vi "Result.vi"(8 "error in (no error)":errorcluster, 10 "Result":T1={"Name"="", "Message"="", "Description"="", "Status"=enum."Passed", "Result Type"=enum."Case", "Execution Time"=0.0}, 11 "Test Result Tree V2 in":refnum<class "Test Result Tree V2.lvclass">) -> (0 "error out":errorcluster)   [LabVIEW 2020, in "Test Result Tree V2.lvclass"]
uses:
  Test Result Tree V2.lvclass
  C:/Git/astemes-lunit/source/Rewrite Project/Deprecated/Test Tree/Test Tree.lvclass
  Result/Result.ctl
  Result/Status.ctl
  Result/Type.ctl
  Test Tree/Test Tree.lvclass/Test Tree.ctl
  Utilities/Status to Glyph.vi
  Test Tree/Test Tree.lvclass
  Result/Result.lvlib
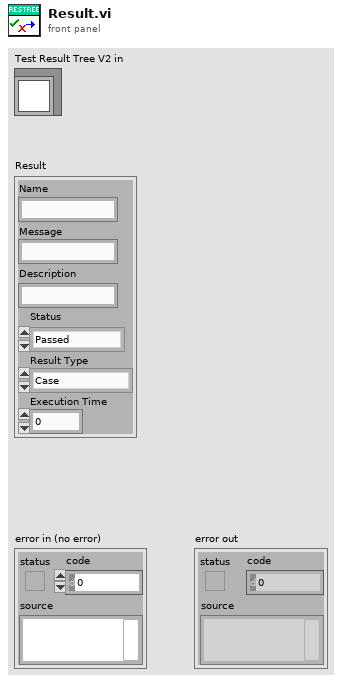
[diagram p1: front panel]
types:
  T1 = typedef "Result.lvlib/Result.ctl" = cluster{"Name":string, "Message":string, "Description":string, "Status":T2, "Result Type":T3, "Execution Time":dbl}
  T2 = typedef "Result.lvlib/Status.ctl" = enum16{"", "Passed", "Failed", "Error", "Skipped", "Setup Error", "Broken", "Teardown Error"}
  T3 = typedef "Result.lvlib/Type.ctl" = enum16{"Method", "Case", "Suite", "Pass", "Fail", "Skip", "Pass if", "Fail if", "Pass if Error", "Fail if Error", "Pass if Equal", "Fail if Equal"}
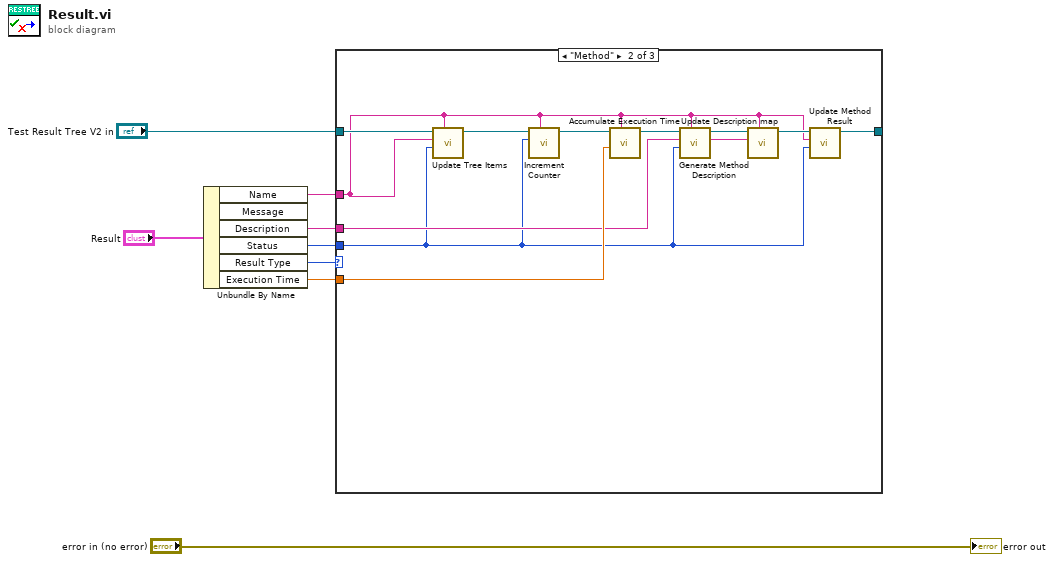
[diagram p0: block diagram]
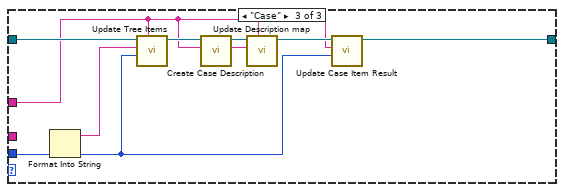
[diagram p3: hidden frame]
diagram:
  n1 = Unbundle By Name("Result") -> ("Name"=w5:string, "Description"=w1:string, "Status"=w4:T2, "Result Type"=w7:T3, "Execution Time"=w3:dbl)  [unwired: 1 out]
  n2 = case shown="\"Method\"" w7 {
    tunnel: "Test Result Tree V2 in" -> [w9 w19 w30]
    tunnel: [w9 w16 w24] -> _
    tunnel: w5 -> [_ w11 w23]
    tunnel: w4 -> [_ w10 w22]
    tunnel: w3 -> [_ w18 _]
    tunnel: w1 -> [_ w12 _]
    frame Default {
    }
    frame "Method" {
      n3 = call "Update Tree Items.vi"("Item"=w11, "Status"=w10, "Child Text"=w11, "Test Tree In"=w19) -> ("Test Tree Out"=w20:refnum<class "Test Result Tree V2.lvclass">)  [unwired: 7 in]
      n4 = call "Increment Counter.vi"("Method Name"=w11, "Status"=w10, "Test Result Tree V2 in"=w20) -> ("Test Result Tree V2 out"=w21:refnum<class "Test Result Tree V2.lvclass">)  [unwired: 8 in]
      n5 = call "Accumulate Execution Time.vi"("Method Name"=w11, "Execution Time"=w18, "Test Result Tree V2 in"=w21) -> ("Test Result Tree V2 out"=w15:refnum<class "Test Result Tree V2.lvclass">)  [unwired: 8 in]
      n6 = call "Generate Method Description.vi"("Name"=w11, "Status"=w10, "Descirption"=w12, "Test Tree In"=w15) -> ("Description"=w13:string, "Test Tree Out"=w14:refnum<class "Test Result Tree V2.lvclass">)  [unwired: 6 in]
      n7 = call "Update Description map.vi"("Item"=w11, "Description"=w13, "Test Tree In"=w14) -> ("Test Tree Out"=w17:refnum<class "Test Result Tree V2.lvclass">)  [unwired: 8 in]
      n8 = call "Update Method Result.vi"("Status"=w10, "Case"=w11, "Test Tree In"=w17) -> ("Test Tree Out"=w16:refnum<class "Test Result Tree V2.lvclass">)  [unwired: 8 in]
    }
    frame "Case" {
      n9 = Format Into String(w22) -> (resulting string=w29:string)  [unwired: 3 in, 1 out]
      n10 = call "Update Tree Items.vi"("Item"=w23, "Status"=w22, "Child Text"=w29, "Test Tree In"=w30) -> ("Test Tree Out"=w28:refnum<class "Test Result Tree V2.lvclass">)  [unwired: 7 in]
      n11 = call "Create Case Description.vi"("Case"=w23, "Test Result Tree V2 in"=w28) -> ("Description"=w26:string, "Test Result Tree V2 in 2"=w27:refnum<class "Test Result Tree V2.lvclass">)  [unwired: 8 in]
      n12 = call "Update Description map.vi"("Item"=w23, "Description"=w26, "Test Tree In"=w27) -> ("Test Tree Out"=w25:refnum<class "Test Result Tree V2.lvclass">)  [unwired: 8 in]
      n13 = call "Update Case Item Result.vi"("Status"=w22, "Test Case"=w23, "Test Result Tree V2 in"=w25) -> ("Test Result Tree V2 out"=w24:refnum<class "Test Result Tree V2.lvclass">)  [unwired: 8 in]
    }
  }
  "error out" <- "error in (no error)"
